vi "Set_Daxsonics_3Pulsers.vi"(8 "Number of Channels":i32=5, 9 "Daxsonics Settings":T1={"Freq (MHz) "=20, "Voltage (V)"=0, "Gain (dB)"=22} {"Freq (MHz)" items=["50"=50, "45"=45, "40"=40, "35"=35, "30"=30, "25"=25, "20"=20, "18"=18, "17"=17, "16"=16, "15"=15, "14"=14, "12"=12, "10"=10, "8"=8, "6"=6, "5"=5, "4"=4]; "Voltage (V)" items=["190"=190, "180"=180, "170"=170, "160"=160, "150"=150, "140"=140, "130"=130, "120"=120, "110"=110, "100"=100, "95"=95, "90"=90, "85"=85, "80"=80, "75"=75, "70"=70, "65"=65, "60"=60, "55"=55, "50"=50, "45"=45, "40"=40, "35"=35, "30"=30, "25"=25, "20"=20, "15"=15, "10"=10, "5"=5, "0"=0]; "Gain (dB)" items=["67"=67, "64"=64, "61"=61, "58"=58, "55"=55, "52"=52, "49"=49, "46"=46, "43"=43, "40"=40, "37"=37, "34"=34, "31"=31, "28"=28, "25"=25, "22"=22]}) -> ()   [LabVIEW 2022 SP3]
doc: "This application VI allows the user to set the desired parameters in the \n5800 / 5900 P / R. just select thevalues that you want to set the instrument to from the 5800 / 5900 user interface and click on the send to 5800 button."
uses:
  -DaxSubroutines/Dax_Control_Cluster.ctl
  PulserGlobals.vi
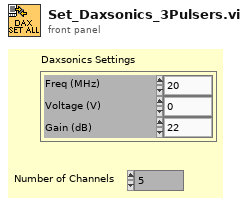
[diagram p1: front panel]
types:
  T1 = typedef "Dax_Control_Cluster.ctl" = cluster{"Freq (MHz) ":u16, "Voltage (V)":u16, "Gain (dB)":u16}
  T2 = typedef "Daxsonics_Pulsers.ctl" = enum16{"BP1", "BP2_A", "BP2_B", "10ERS8", "New2021"}
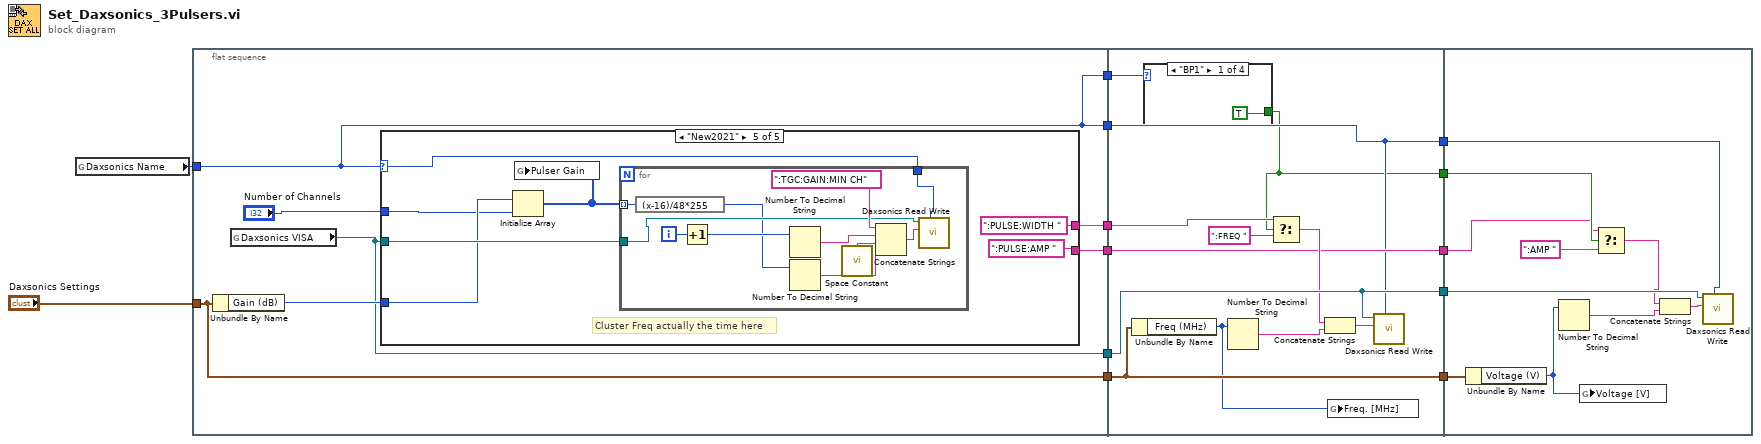
[diagram p0: block diagram]
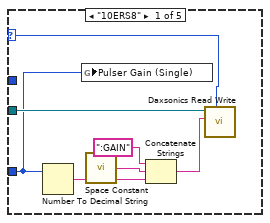
[diagram p2: hidden frame]
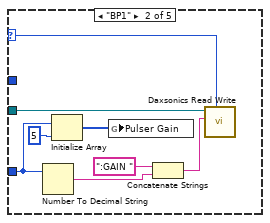
[diagram p3: hidden frame]
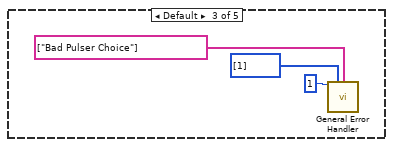
[diagram p4: hidden frame]
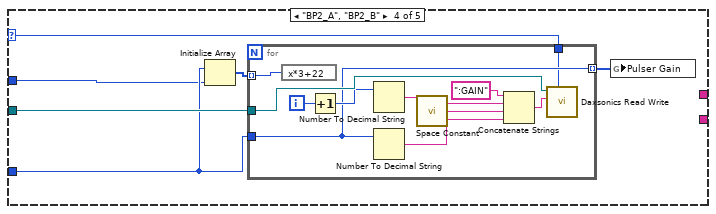
[diagram p5: hidden frame]
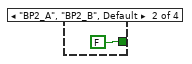
[diagram p6: hidden frame]
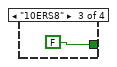
[diagram p7: hidden frame]
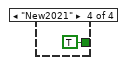
[diagram p8: hidden frame]
diagram:
  n1 = global read "PulserGlobals.vi" "Daxsonics Name"() -> (w8:T2)
  n2 = flat-sequence {
    tunnel: [w18] -> w12
    tunnel: "Daxsonics Settings" -> [w20]
    tunnel: [w20] -> w11
    tunnel: w8 -> [w14]
    tunnel: [w16] -> w6
    tunnel: [w15] -> w4
    tunnel: [w14] -> w3
    tunnel: [w14] -> w1
    tunnel: [w84] -> w13
    tunnel: w12 -> [w84]
    tunnel: w11 -> [w82]
    tunnel: [w82] -> w10
    tunnel: [w74] -> w7
    tunnel: w6 -> [w79]
    tunnel: [w78] -> w5
    tunnel: w4 -> [w78]
    tunnel: w3 -> [w76]
    tunnel: [w76] -> w2
    tunnel: w1 -> [w75]
    tunnel: w13 -> [w97]
    tunnel: w10 -> [w96]
    tunnel: w7 -> [w92]
    tunnel: w5 -> [w91]
    tunnel: w2 -> [w90]
    frame #0 {
      n3 = Unbundle By Name(w20) -> ("Gain (dB)"=w19:u16)
      n4 = global read "PulserGlobals.vi" "Daxsonics VISA"() -> (w18:refnum<visa-resource-name>)
      n5 = case shown="\"New2021\"" w14 {
        selector: w14 -> [w21 w28 _ w39 w56]
        tunnel: w18 -> [w23 w30 _ w43 w62]
        tunnel: w19 -> [w22 w31 _ w42 w61]
        tunnel: "Number of Channels" -> [_ _ _ w40 w60]
        tunnel: [_ _ _ _ ":PULSE:WIDTH " ("string")] -> w16
        tunnel: [_ _ _ _ ":PULSE:AMP " ("string")] -> w15
        frame "10ERS8" {
          n6 = Number To Decimal String(number=w22) -> (decimal integer string=w27:string)  [unwired: 1 in]
          n7 = global write "PulserGlobals.vi" "Pulser Gain (Single)"(w22) -> ()
          n8 = call <vilib>:"Space Constant.vi"() -> ("String"=w24:string)
          n9 = Concatenate Strings(":GAIN" ("string"), w24, w27) -> (w26:string)
          n10 = call "Daxsonics Read Write.vi"("Daxsonics Name"=w21, "write buffer"=w26, "VISA resource name"=w23) -> ()  [unwired: 6 in, 3 out]
        }
        frame "BP1" {
          n11 = Number To Decimal String(number=w31) -> (decimal integer string=w34:string)  [unwired: 1 in]
          n12 = Initialize Array(w31, 5 ("dimension size")) -> (w29:u16[])
          n13 = global write "PulserGlobals.vi" "Pulser Gain"(w29) -> ()
          n14 = Concatenate Strings(":GAIN " ("string"), w34) -> (w32:string)
          n15 = call "Daxsonics Read Write.vi"("Daxsonics Name"=w28, "write buffer"=w32, "VISA resource name"=w30) -> ()  [unwired: 6 in, 3 out]
        }
        frame Default {
          n16 = call <vilib>:"General Error Handler.vi"("[error code] (0)"=1, "[user-defined codes]"=i32[] [1], "[user-defined descriptions]"=string[] ["Bad Pulser Choice"]) -> ()  [unwired: 8 in, 5 out]
        }
        frame "BP2_A", "BP2_B" {
          n17 = Initialize Array(w42, w40) -> (w44:u16[])
          n18 = for {
            tunnel: w43 -> [w52]
            tunnel: w44 -> [w47] mode=indexing
            tunnel: [w46] -> w41 mode=indexing
            tunnel: w42 -> [w46]
            tunnel: w39 -> [w45]
            i -> [w51]
            n19 = expression code="x*3+22"(w47) -> ()  [unwired: 1 out]
            n20 = Increment(x=w51) -> (x+1=w48:i32)
            n21 = Number To Decimal String(number=w48) -> (decimal integer string=w50:string)  [unwired: 1 in]
            n22 = Number To Decimal String(number=w46) -> (decimal integer string=w55:string)  [unwired: 1 in]
            n23 = call <vilib>:"Space Constant.vi"() -> ("String"=w49:string)
            n24 = Concatenate Strings(":GAIN" ("string"), w50, w49, w55) -> (w54:string)
            n25 = call "Daxsonics Read Write.vi"("Daxsonics Name"=w45, "write buffer"=w54, "VISA resource name"=w52) -> ()  [unwired: 6 in, 3 out]
          }
          n26 = global write "PulserGlobals.vi" "Pulser Gain"(w41) -> ()
        }
        frame "New2021" {
          # "Cluster Freq actually the time here"
          n27 = Initialize Array(w61, w60) -> (w57:u16[])
          n28 = global write "PulserGlobals.vi" "Pulser Gain"(w57) -> ()
          n29 = for {
            tunnel: w62 -> [w71]
            tunnel: w57 -> [w66] mode=indexing
            tunnel: w56 -> [w63]
            i -> [w70]
            n30 = expression code="(x-16)/48*255"(w66) -> (w65:u16)
            n31 = Increment(x=w70) -> (x+1=w67:i32)
            n32 = Number To Decimal String(number=w67) -> (decimal integer string=w69:string)  [unwired: 1 in]
            n33 = Number To Decimal String(number=w65) -> (decimal integer string=w64:string)  [unwired: 1 in]
            n34 = call <vilib>:"Space Constant.vi"() -> ("String"=w68:string)
            n35 = Concatenate Strings(":TGC:GAIN:MIN CH" ("string"), w69, w68, w64) -> (w73:string)
            n36 = call "Daxsonics Read Write.vi"("Daxsonics Name"=w63, "write buffer"=w73, "VISA resource name"=w71) -> ()  [unwired: 6 in, 3 out]
          }
        }
      }
    }
    frame #1 {
      n37 = Unbundle By Name(w82) -> ("Freq (MHz)"=w77:u16)
      n38 = case shown="\"BP1\"" w75 {
        tunnel: [TRUE ("Enable Termination\nChar (T)") FALSE ("Enable Termination\nChar (T)") FALSE ("Enable Termination\nChar (T)") TRUE ("CR on Write?")] -> w74
        frame "BP1" {
        }
        frame "BP2_A", "BP2_B", Default {
        }
        frame "10ERS8" {
        }
        frame "New2021" {
        }
      }
      n39 = Number To Decimal String(number=w77) -> (decimal integer string=w83:string)  [unwired: 1 in]
      n40 = Select(t=w79, s=w74, f=":FREQ " ("string")) -> (s? t:f=w80:string)
      n41 = Concatenate Strings(w80, w83) -> (w85:string)
      n42 = global write "PulserGlobals.vi" "Freq. [MHz]"(w77) -> ()
      n43 = call "Daxsonics Read Write.vi"("Daxsonics Name"=w76, "write buffer"=w85, "VISA resource name"=w84) -> ()  [unwired: 6 in, 3 out]
    }
    frame #2 {
      n44 = Unbundle By Name(w96) -> ("Voltage (V)"=w95:u16)
      n45 = Number To Decimal String(number=w95) -> (decimal integer string=w99:string)  [unwired: 1 in]
      n46 = global write "PulserGlobals.vi" "Voltage [V]"(w95) -> ()
      n47 = Select(t=w91, s=w92, f=":AMP " ("string")) -> (s? t:f=w93:string)
      n48 = Concatenate Strings(w93, w99) -> (w98:string)
      n49 = call "Daxsonics Read Write.vi"("Daxsonics Name"=w90, "write buffer"=w98, "VISA resource name"=w97) -> ()  [unwired: 6 in, 3 out]
    }
  }
